vi "Emballage check code lu_MEDIC.vi"(0 "pièce en stock (testée et non emballée)":string[](array[string]), 1 "Quantité du lot de livraison":string="25", 2 "son code lu incorrect":path=path "\\\\Plz-inf-nas\\medic/PARAMETRES_TESTS/PROD_Data-Admin/Utopia - Erreur.WAV", 3 "n°commande":string="R03770/08-02.01.01", 5 "tableau des paramètres de la valve":string[](array[string])=["12-216C-04521 EQIFIL 104mA 230ohm", "1121058500", "AASSIIII", "25", "BPI", "n", "o"], 7 "tab pcs emballées historique":string[][](array[string]), 9 "chaîne lue par le lecteur IN":string="112105740008010105", 11 "tab pcs déjà emballées (histo+actu)":string[](array[string]), 12 "son code lu correct":path=path "\\\\Plz-inf-nas\\medic/PARAMETRES_TESTS/PROD_Data-Admin/lazer.wav", 13 "n° lot à scanner":string="****") -> (4 "largeur index":i16=4, 6 "Date production de la piéce":string="ZF", 8 "chaîne lue par le lecteur OUT":string="8411848-12ARZF-0005", 10 "Arrêter la série (T)":bool, 14 "offset sur code bar début index":i16=15, 15 "Paramètres OK(=> T)":bool=TRUE)   [LabVIEW 2020]
uses:
  Instance           3 31Saved   Emballage check code lu .vi
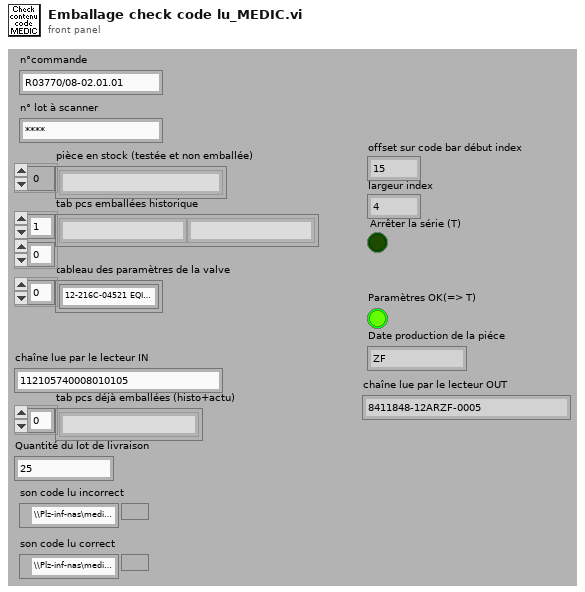
[diagram p1: front panel]
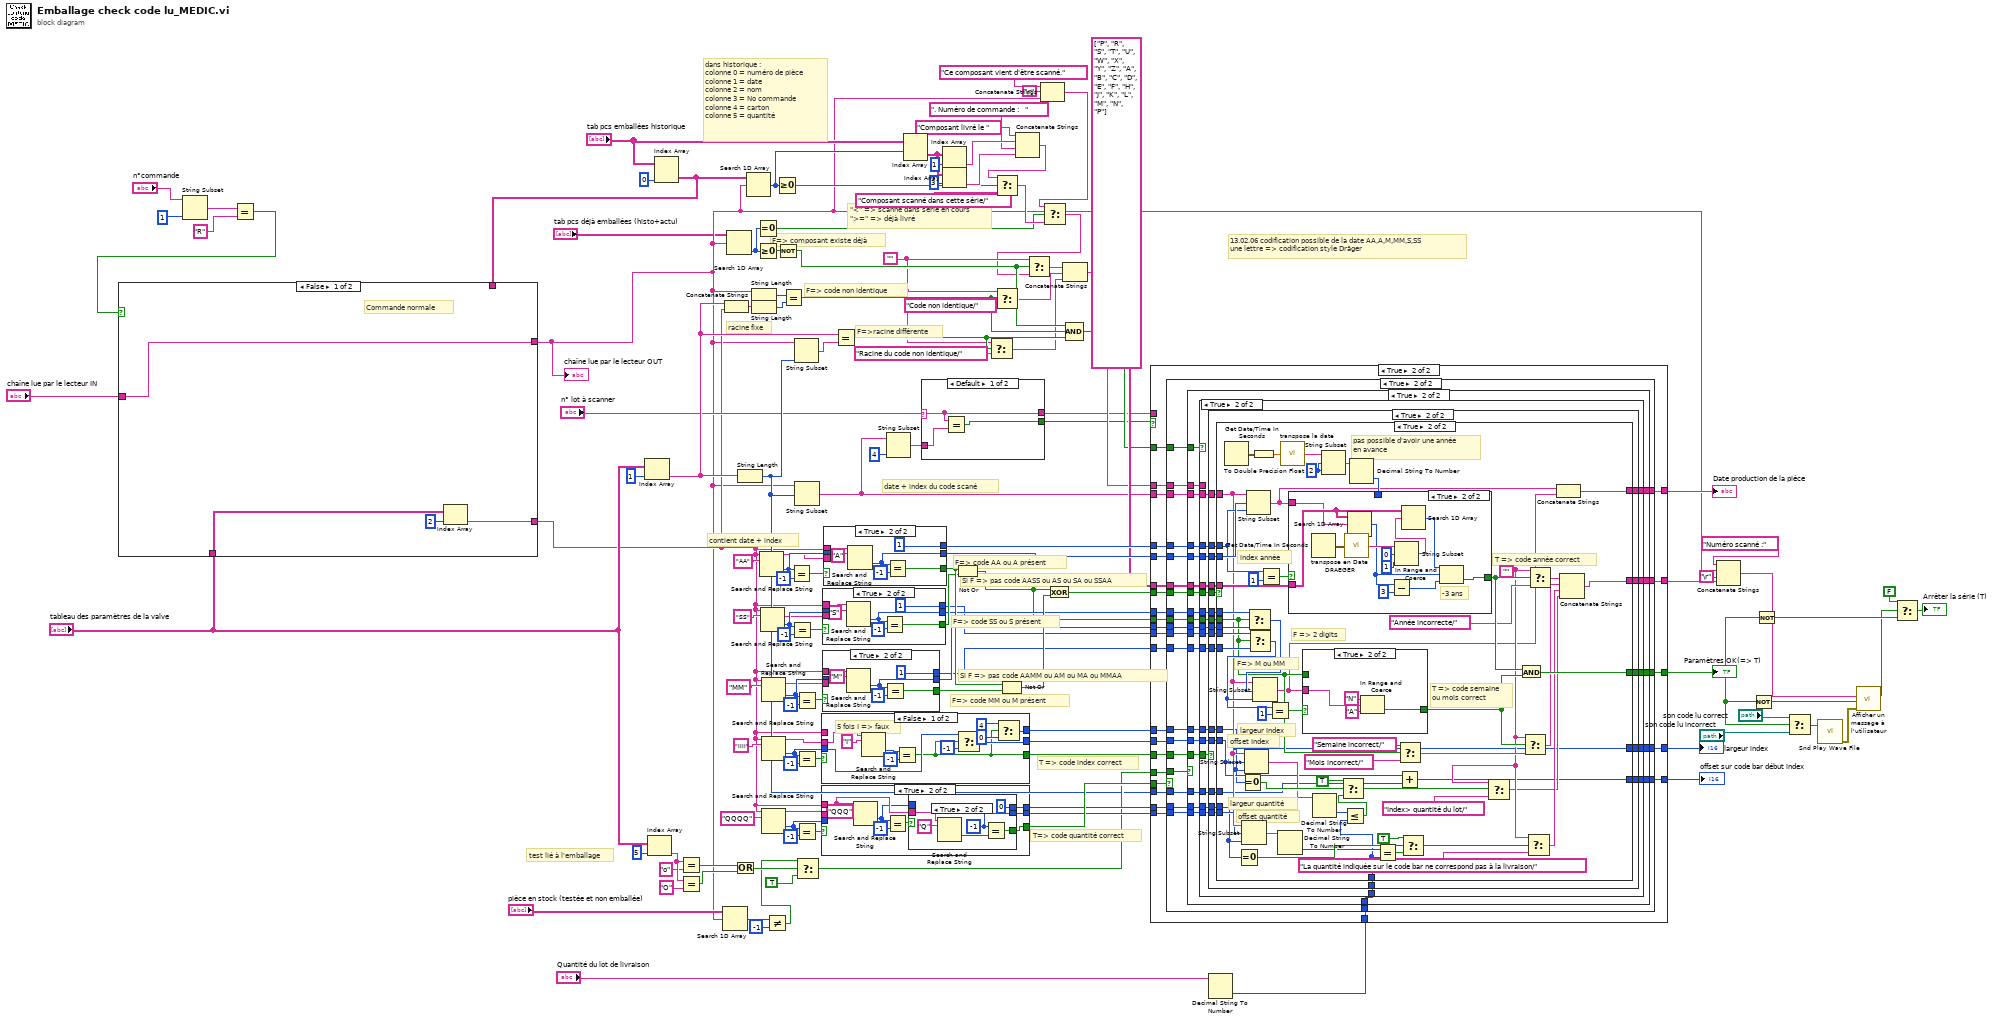
[diagram p0: block diagram]
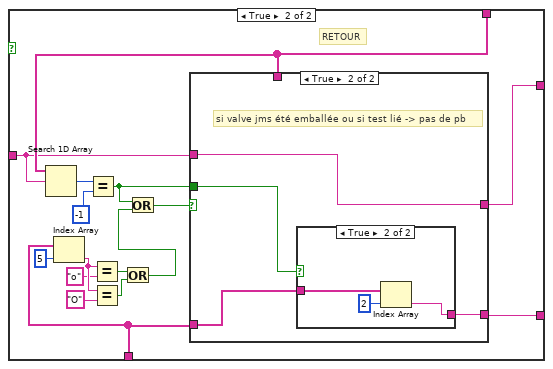
[diagram p2: hidden frame]
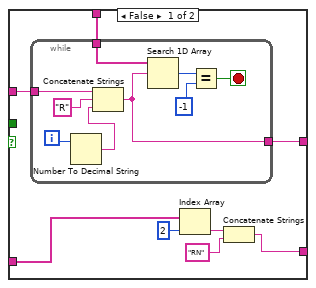
[diagram p3: hidden frame]
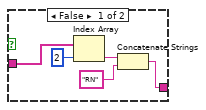
[diagram p4: hidden frame]
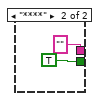
[diagram p5: hidden frame]
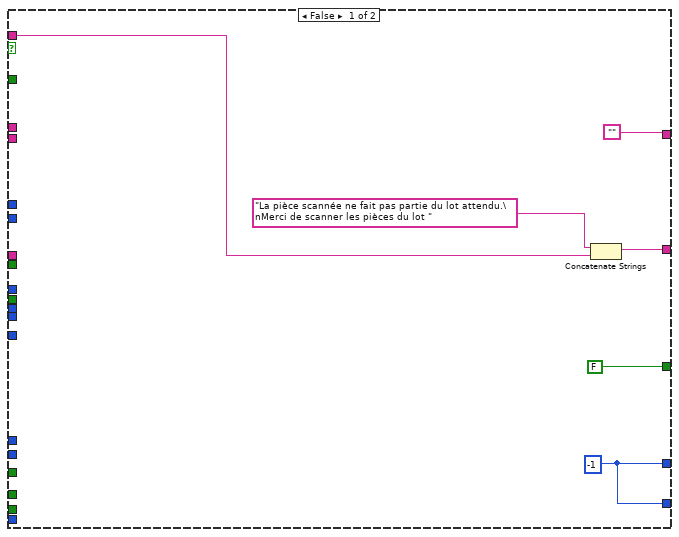
[diagram p6: hidden frame]
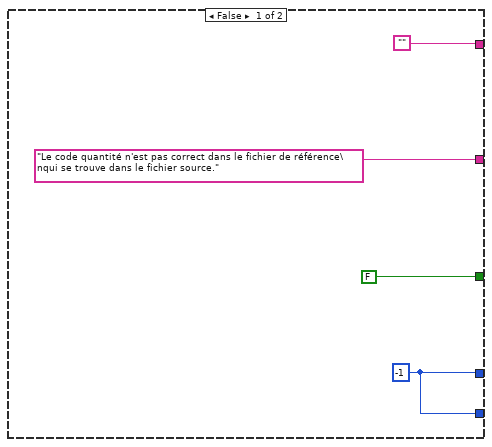
[diagram p7: hidden frame]
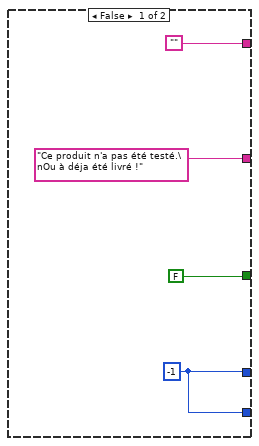
[diagram p8: hidden frame]
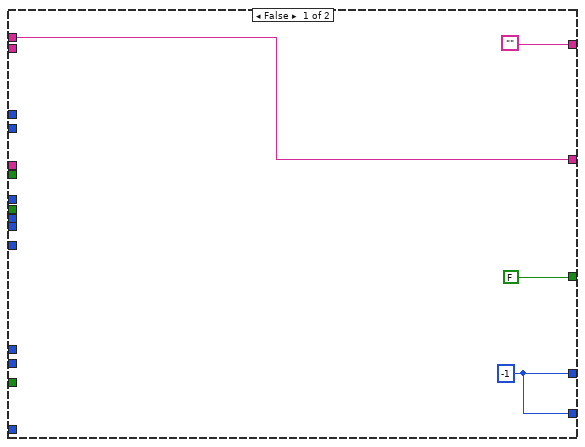
[diagram p9: hidden frame]
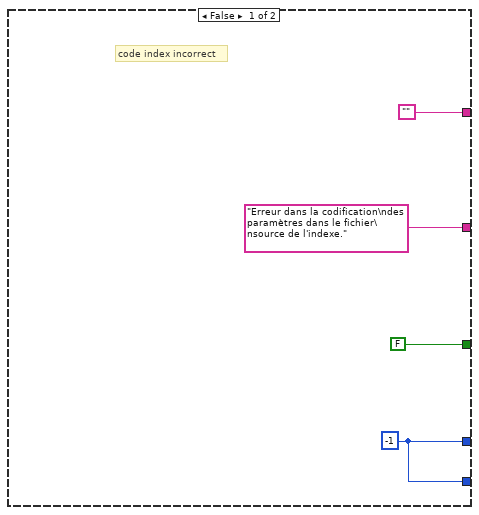
[diagram p10: hidden frame]
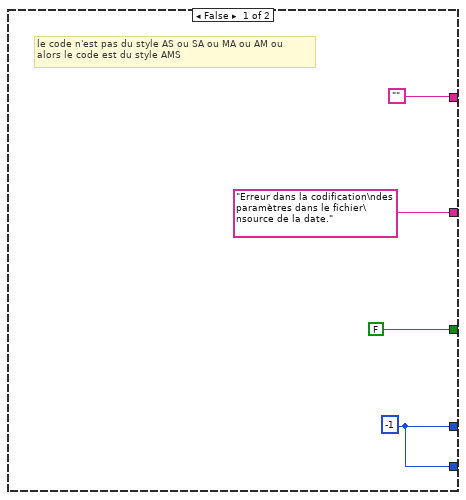
[diagram p11: hidden frame]
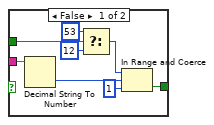
[diagram p12: hidden frame]
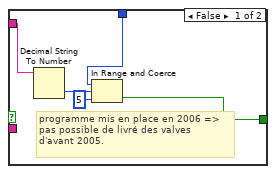
[diagram p13: hidden frame]
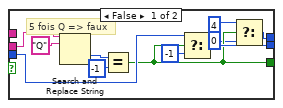
[diagram p14: hidden frame]
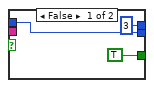
[diagram p15: hidden frame]
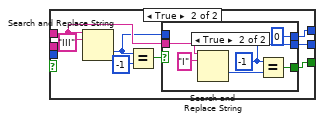
[diagram p16: hidden frame]
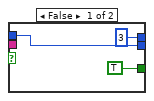
[diagram p17: hidden frame]
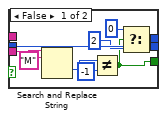
[diagram p18: hidden frame]
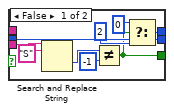
[diagram p19: hidden frame]
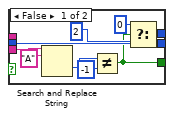
[diagram p20: hidden frame]
diagram:
  w91 = ""
  # "dans historique :\ncolonne 0 = numéro de pièce\ncolonne 1 = date\ncolonne 2 = nom\ncolonne 3 = No commande\ncolonne 4 = carton\ncolonne 5 = quantité"
  # "\"<\" => scanné dans série en cours\n\">=\" => déjà livré"
  # "T=> code quantité correct"
  # "test lié à l'emballage"
  # "Si F => pas code AASS ou AS ou SA ou SSAA"
  # "Si F => pas code AAMM ou AM ou MA ou MMAA"
  # "F=> code MM ou M présent"
  # "F=> code SS ou S présent"
  # "F=> code AA ou A présent"
  # "T => code index correct"
  # "13.02.06 codification possible de la date AA,A,M,MM,S,SS\nune lettre => codification style Dräger"
  # "date + index du code scané"
  # "contient date + index"
  # "racine fixe"
  # "F=> composant existe déjà"
  # "F=> code non identique"
  # "F=>racine différente"
  n1 = String Subset(string="n°commande", length (rest)=1 ("longueur (reste)")) -> (substring=w11:string)  [unwired: 1 in]
  n2 = Equal?(x=w11, y="R" ("expression régulière")) -> (x = y?=w10:bool)
  n3 = Index Array(array="tableau des paramètres de la valve", index=1) -> (element=w127:string)
  n4 = Index Array(array="tableau des paramètres de la valve", index=5) -> (element=w84:string)
  n5 = Index Array(array="tab pcs emballées historique", index (col)=0) -> (element=w1:string[])  [unwired: 1 in]
  n6 = case shown="False" w10 {
    tunnel: "chaîne lue par le lecteur IN" -> [w136 w149]
    tunnel: [w136 w148] -> w3
    tunnel: w1 -> [_ w150]
    tunnel: "tableau des paramètres de la valve" -> [w134 w138]
    tunnel: [w133 w139] -> w4
    frame False {
      # "Commande normale"
      n7 = Index Array(array=w134, index=2) -> (element=w133:string)
    }
    frame True {
      # "RETOUR"
      n8 = Search 1D Array(1D array=w150, element=w149) -> (index of element=w151:i32)  [unwired: 1 in]
      n9 = Index Array(array=w138, index=5) -> (element=w144:string)
      n10 = Equal?(x=w151, y=-1) -> (x = y?=w137:bool)
      n11 = Equal?(x=w144, y="o") -> (x = y?=w145:bool)
      n12 = Equal?(x=w144, y="O") -> (x = y?=w141:bool)
      n13 = Or(x=w145, y=w141) -> (x .or. y?=w140:bool)
      n14 = Or(x=w137, y=w140) -> (x .or. y?=w147:bool)
      n15 = case shown="True" w147 {
        tunnel: w150 -> [w160 _]
        tunnel: w149 -> [w159 w173]
        tunnel: [w158 w173] -> w148
        tunnel: [w154 w172] -> w139
        tunnel: w138 -> [w153 w171]
        tunnel: w137 -> [_ w170]
        frame False {
          n16 = while {
            tunnel: w160 -> [w168]
            tunnel: w159 -> [w167]
            tunnel: [w161] -> w158
            i -> [w165]
            stop <- w162 stop-if-true
            n17 = Number To Decimal String(number=w165) -> (decimal integer string=w166:string)  [unwired: 1 in]
            n18 = Concatenate Strings(w167, "R" ("expression régulière"), w166) -> (w161:string)
            n19 = Search 1D Array(1D array=w168, element=w161) -> (index of element=w164:i32)  [unwired: 1 in]
            n20 = Equal?(x=w164, y=-1) -> (x = y?=w162:bool)
          }
          n21 = Index Array(array=w153, index=2) -> (element=w156:string)
          n22 = Concatenate Strings(w156, "RN" ("chaîne")) -> (w154:string)
        }
        frame True {
          # "si valve jms été emballée ou si test lié -> pas de pb"
          n23 = case shown="True" w170 {
            tunnel: [w174 w180] -> w172
            tunnel: w171 -> [w177 w179]
            frame False {
              n24 = Index Array(array=w177, index=2) -> (element=w176:string)
              n25 = Concatenate Strings(w176, "RN" ("chaîne")) -> (w174:string)
            }
            frame True {
              n26 = Index Array(array=w179, index=2) -> (element=w180:string)
            }
          }
        }
      }
    }
  }
  "chaîne lue par le lecteur OUT" <- w3
  n27 = Equal?(x=w84, y="o") -> (x = y?=w85:bool)
  n28 = Equal?(x=w84, y="O") -> (x = y?=w81:bool)
  n29 = Search 1D Array(1D array="pièce en stock (testée et non emballée)", element=w3) -> (index of element=w62:i32)  [unwired: 1 in]
  n30 = Concatenate Strings(w127, w4) -> (w132:string)
  n31 = Search 1D Array(1D array="tab pcs déjà emballées (histo+actu)", element=w3) -> (index of element=w24:i32)  [unwired: 1 in]
  n32 = Or(x=w85, y=w81) -> (x .or. y?=w60:bool)
  n33 = String Length(string=w127) -> (length=w55:i32)
  n34 = Search 1D Array(1D array=w1, element=w3) -> (index of element=w25:i32)  [unwired: 1 in]
  n35 = String Length(string=w3) -> (length=w131:i32)
  n36 = String Length(string=w132) -> (length=w130:i32)
  n37 = Equal To 0?(x=w24) -> (x = 0?=w21:bool)
  n38 = Greater Or Equal To 0?(x=w24) -> (x >= 0?=w95:bool)
  n39 = Search and Replace String(input string=w4, search string="AA") -> (result string=w79:string, offset past replacement=w114:i32)  [unwired: 6 in, 2 out]
  n40 = Search and Replace String(input string=w4, search string="SS") -> (result string=w64:string, offset past replacement=w113:i32)  [unwired: 6 in, 2 out]
  n41 = Search and Replace String(input string=w4, search string="MM") -> (result string=w63:string, offset past replacement=w112:i32)  [unwired: 6 in, 2 out]
  n42 = Search and Replace String(input string=w4, search string="IIII") -> (result string=w80:string, offset past replacement=w73:i32)  [unwired: 6 in, 2 out]
  n43 = Search and Replace String(input string=w4, search string="QQQQ") -> (result string=w71:string, offset past replacement=w70:i32)  [unwired: 6 in, 2 out]
  n44 = Not Equal?(x=w62, y=-1) -> (x != y?=w56:bool)
  n45 = Greater Or Equal To 0?(x=w25) -> (x >= 0?=w31:bool)
  n46 = Not(x=w95) -> (.not. x?=w94:bool)
  n47 = Equal?(x=w131, y=w130) -> (x = y?=w96:bool)
  n48 = Equal?(x=w114, y=-1) -> (x = y?=w119:bool)
  n49 = Equal?(x=w113, y=-1) -> (x = y?=w120:bool)
  n50 = String Subset(string=w3, length (rest)=w55) -> (substring=w128:string)  [unwired: 1 in]
  n51 = String Subset(string=w3, offset (0)=w55) -> (substring=w14:string)  [unwired: 1 in]
  n52 = Equal?(x=w112, y=-1) -> (x = y?=w118:bool)
  n53 = Equal?(x=w73, y=-1) -> (x = y?=w115:bool)
  n54 = Equal?(x=w70, y=-1) -> (x = y?=w65:bool)
  n55 = Select(t=w56, s=w60, f=TRUE) -> (s? t:f=w58:bool)
  n56 = case shown="False" w115 {
    tunnel: w4 -> [_ w197]
    tunnel: [w183 w196] -> w74
    tunnel: w80 -> [w189 _]
    tunnel: w73 -> [w188 _]
    tunnel: [w186 w194] -> w72
    tunnel: [w182 w193] -> w67
    frame False {
      # "5 fois I => faux"
      n57 = Search and Replace String(input string=w189, search string="I") -> (offset past replacement=w190:i32)  [unwired: 6 in, 3 out]
      n58 = Equal?(x=w190, y=-1) -> (x = y?=w183:bool)
      n59 = Select(t=w188, s=w183, f=-1) -> (s? t:f=w186:i32)
      n60 = Select(t=4, s=w183, f=0) -> (s? t:f=w182:i32)
    }
    frame True {
      n61 = Search and Replace String(input string=w197, search string="III") -> (offset past replacement=w195:i32)  [unwired: 6 in, 3 out]
      n62 = Equal?(x=w195, y=-1) -> (x = y?=w198:bool)
      n63 = case shown="True" w198 {
        tunnel: w197 -> [_ w208]
        tunnel: [TRUE w206] -> w196
        tunnel: w195 -> [w202 _]
        tunnel: [w202 w205] -> w194
        tunnel: [3 0] -> w193
        frame False {
        }
        frame True {
          w205 = -1
          n64 = Search and Replace String(input string=w208, search string="I") -> (offset past replacement=w207:i32)  [unwired: 6 in, 3 out]
          n65 = Equal?(x=w205, y=w207) -> (x = y?=w206:bool)
        }
      }
    }
  }
  n66 = case shown="True" w65 {
    tunnel: w4 -> [_ w225]
    tunnel: [w213 w224] -> w69
    tunnel: w71 -> [w217 _]
    tunnel: w70 -> [w216 _]
    tunnel: [w214 w222] -> w68
    tunnel: [w210 w221] -> w66
    frame False {
      # "5 fois Q => faux"
      n67 = Search and Replace String(input string=w217, search string="Q") -> (offset past replacement=w218:i32)  [unwired: 6 in, 3 out]
      n68 = Equal?(x=w218, y=-1) -> (x = y?=w213:bool)
      n69 = Select(t=w216, s=w213, f=-1) -> (s? t:f=w214:i32)
      n70 = Select(t=4, s=w213, f=0) -> (s? t:f=w210:i32)
    }
    frame True {
      n71 = Search and Replace String(input string=w225, search string="QQQ") -> (offset past replacement=w223:i32)  [unwired: 6 in, 3 out]
      n72 = Equal?(x=w223, y=-1) -> (x = y?=w226:bool)
      n73 = case shown="True" w226 {
        tunnel: w225 -> [_ w236]
        tunnel: [TRUE w234] -> w224
        tunnel: w223 -> [w230 _]
        tunnel: [w230 w233] -> w222
        tunnel: [3 0] -> w221
        frame False {
        }
        frame True {
          w233 = -1
          n74 = Search and Replace String(input string=w236, search string="Q") -> (offset past replacement=w235:i32)  [unwired: 6 in, 3 out]
          n75 = Equal?(x=w233, y=w235) -> (x = y?=w234:bool)
        }
      }
    }
  }
  n76 = case shown="True" w118 {
    tunnel: w4 -> [_ w252]
    tunnel: [w239 w249] -> w111
    tunnel: [w246 w248] -> w103
    tunnel: w112 -> [w246 _]
    tunnel: [w241 1] -> w100
    tunnel: w63 -> [w242 _]
    frame False {
      n77 = Search and Replace String(input string=w242, search string="M") -> (offset past replacement=w245:i32)  [unwired: 6 in, 3 out]
      n78 = Not Equal?(x=w245, y=-1) -> (x != y?=w239:bool)
      n79 = Select(t=0, s=w239, f=2) -> (s? t:f=w241:i32)
    }
    frame True {
      n80 = Search and Replace String(input string=w252, search string="M") -> (offset past replacement=w248:i32)  [unwired: 6 in, 3 out]
      n81 = Equal?(x=w248, y=-1) -> (x = y?=w249:bool)
    }
  }
  n82 = case shown="True" w120 {
    tunnel: w4 -> [_ w267]
    tunnel: w113 -> [w261 _]
    tunnel: [w261 w264] -> w104
    tunnel: [w253 w263] -> w109
    tunnel: [w256 1] -> w101
    tunnel: w64 -> [w257 _]
    frame False {
      n83 = Search and Replace String(input string=w257, search string="S") -> (offset past replacement=w258:i32)  [unwired: 6 in, 3 out]
      n84 = Not Equal?(x=w258, y=-1) -> (x != y?=w253:bool)
      n85 = Select(t=0, s=w253, f=2) -> (s? t:f=w256:i32)
    }
    frame True {
      n86 = Search and Replace String(input string=w267, search string="S") -> (offset past replacement=w264:i32)  [unwired: 6 in, 3 out]
      n87 = Equal?(x=w264, y=-1) -> (x = y?=w263:bool)
    }
  }
  n88 = case shown="True" w119 {
    tunnel: w4 -> [_ w281]
    tunnel: w114 -> [w276 _]
    tunnel: [w276 w279] -> w106
    tunnel: [w268 w278] -> w110
    tunnel: [w271 1] -> w105
    tunnel: w79 -> [w274 _]
    frame False {
      n89 = Search and Replace String(input string=w274, search string="A") -> (offset past replacement=w272:i32)  [unwired: 6 in, 3 out]
      n90 = Not Equal?(x=w272, y=-1) -> (x != y?=w268:bool)
      n91 = Select(t=0, s=w268, f=2) -> (s? t:f=w271:i32)
    }
    frame True {
      n92 = Search and Replace String(input string=w281, search string="A") -> (offset past replacement=w279:i32)  [unwired: 6 in, 3 out]
      n93 = Equal?(x=w279, y=-1) -> (x = y?=w278:bool)
    }
  }
  n94 = Equal?(x=w127, y=w128) -> (x = y?=w97:bool)
  n95 = String Subset(string=w14, length (rest)=4 ("longueur (reste)")) -> (substring=w12:string)  [unwired: 1 in]
  n96 = Index Array(array="tab pcs emballées historique", index (row)=w25) -> (element=w35:string[])  [unwired: 1 in]
  n97 = case shown="Default" "n° lot à scanner" {
    selector: "n° lot à scanner" -> [w283 _]
    tunnel: [w285 TRUE] -> w16
    tunnel: [w283 "" ("n° lot à scanner")] -> w15
    tunnel: w12 -> [w284 _]
    frame Default {
      n98 = Equal?(x=w283, y=w284) -> (x = y?=w285:bool)
    }
    frame "****" {
    }
  }
  n99 = Index Array(array=w35, index=1) -> (element=w39:string)
  n100 = Index Array(array=w35, index=3) -> (element=w34:string)
  n101 = Not Or(1:w109, 2:w110) -> (0:w102:bool)
  n102 = Select(t=w91, s=w97, f="Racine du code non identique/") -> (s? t:f=w88:string)
  n103 = Select(t=w91, s=w96, f="Code non identique/") -> (s? t:f=w89:string)
  n104 = Not Or(1:w111, 2:w110) -> (0:w108:bool)
  n105 = Concatenate Strings("Composant livré le ", w39, ". Numéro de commande :   ", w34) -> (w37:string)
  n106 = Select(t=w37, s=w31, f="Composant scanné dans cette série/") -> (s? t:f=w22:string)
  n107 = Concatenate Strings("Ce composant vient d'être scanné.", "\r", w3) -> (w19:string)
  n108 = Select(t=w19, s=w21, f=w22) -> (s? t:f=w23:string)
  n109 = Select(t=w91, s=w94, f=w23) -> (s? t:f=w90:string)
  n110 = Exclusive Or(1:w108, 2:w102) -> (0:w107:bool)
  n111 = Concatenate Strings(w90, w89, w88) -> (w87:string)
  n112 = Compound Arithmetic op=AND(w94, w96, w97) -> (w98:bool)
  n113 = Decimal String To Number(string="Quantité du lot de livraison") -> (number=w76:i32)  [unwired: 2 in, 1 out]
  n114 = case shown="True" w16 {
    tunnel: w107 -> [_ w319]
    tunnel: w106 -> [_ w318]
    tunnel: w105 -> [_ w317]
    tunnel: w104 -> [_ w316]
    tunnel: w103 -> [_ w315]
    tunnel: w102 -> [_ w314]
    tunnel: w101 -> [_ w313]
    tunnel: w100 -> [_ w312]
    tunnel: w14 -> [_ w311]
    tunnel: string[] ["P", "R", "S", "T", "U", "W", "X", "Y", "Z", "A", "B", "C", "D", "E", "F", "H", "J", "K", "L", "M", "N", "P"] -> [_ w310]
    tunnel: w98 -> [_ w309]
    tunnel: w87 -> [_ w308]
    tunnel: w76 -> [_ w307]
    tunnel: w74 -> [_ w306]
    tunnel: w72 -> [_ w305]
    tunnel: w69 -> [_ w304]
    tunnel: w68 -> [_ w303]
    tunnel: w67 -> [_ w302]
    tunnel: w66 -> [_ w301]
    tunnel: w58 -> [_ w300]
    tunnel: w55 -> [_ w299]
    tunnel: [w288 w298] -> w54
    tunnel: [w288 w297] -> w53
    tunnel: [w291 w296] -> w47
    tunnel: ["" w295] -> w43
    tunnel: [FALSE w294] -> w29
    tunnel: w15 -> [w290 _]
    frame False {
      w288 = -1
      n115 = Concatenate Strings("La pièce scannée ne fait pas partie du lot attendu.\nMerci de scanner les pièces du lot ", w290) -> (w291:string)
    }
    frame True {
      n116 = case shown="True" w304 {
        tunnel: w306 -> [_ w348]
        tunnel: w319 -> [_ w347]
        tunnel: w318 -> [_ w346]
        tunnel: w317 -> [_ w345]
        tunnel: w316 -> [_ w344]
        tunnel: w315 -> [_ w343]
        tunnel: w314 -> [_ w342]
        tunnel: w313 -> [_ w341]
        tunnel: w312 -> [_ w340]
        tunnel: w311 -> [_ w339]
        tunnel: w310 -> [_ w338]
        tunnel: w309 -> [_ w337]
        tunnel: w308 -> [_ w336]
        tunnel: ["Le code quantité n'est pas correct dans le fichier de référence\nqui se trouve dans le fichier source." w335] -> w296
        tunnel: [FALSE w334] -> w294
        tunnel: w300 -> [_ w333]
        tunnel: w307 -> [_ w332]
        tunnel: w305 -> [_ w331]
        tunnel: w303 -> [_ w330]
        tunnel: w302 -> [_ w329]
        tunnel: w301 -> [_ w328]
        tunnel: ["" w327] -> w295
        tunnel: w299 -> [_ w326]
        tunnel: [w320 w325] -> w298
        tunnel: [w320 w324] -> w297
        frame False {
          w320 = -1
        }
        frame True {
          n117 = case shown="True" w333 {
            tunnel: w348 -> [_ w376]
            tunnel: w347 -> [_ w375]
            tunnel: w346 -> [_ w374]
            tunnel: w345 -> [_ w373]
            tunnel: w344 -> [_ w372]
            tunnel: w343 -> [_ w371]
            tunnel: w342 -> [_ w370]
            tunnel: w341 -> [_ w369]
            tunnel: w340 -> [_ w368]
            tunnel: w339 -> [_ w367]
            tunnel: w338 -> [_ w366]
            tunnel: w337 -> [_ w365]
            tunnel: w336 -> [_ w364]
            tunnel: ["Ce produit n'a pas été testé.\nOu à déja été livré !" w363] -> w335
            tunnel: [FALSE w362] -> w334
            tunnel: w332 -> [_ w361]
            tunnel: w331 -> [_ w360]
            tunnel: w330 -> [_ w359]
            tunnel: w329 -> [_ w358]
            tunnel: w328 -> [_ w357]
            tunnel: ["" w356] -> w327
            tunnel: w326 -> [_ w355]
            tunnel: [w349 w354] -> w325
            tunnel: [w349 w353] -> w324
            frame False {
              w349 = -1
            }
            frame True {
              n118 = case shown="True" w365 {
                tunnel: w376 -> [_ w402]
                tunnel: w375 -> [_ w401]
                tunnel: w374 -> [_ w400]
                tunnel: w373 -> [_ w399]
                tunnel: w372 -> [_ w398]
                tunnel: w371 -> [_ w397]
                tunnel: w370 -> [_ w396]
                tunnel: w369 -> [_ w395]
                tunnel: w368 -> [_ w394]
                tunnel: w367 -> [_ w393]
                tunnel: w366 -> [_ w392]
                tunnel: w364 -> [w380 _]
                tunnel: [w380 w390] -> w363
                tunnel: [FALSE w391] -> w362
                tunnel: w361 -> [_ w389]
                tunnel: w360 -> [_ w388]
                tunnel: w359 -> [_ w387]
                tunnel: w358 -> [_ w386]
                tunnel: w357 -> [_ w385]
                tunnel: ["" w384] -> w356
                tunnel: w355 -> [_ w383]
                tunnel: [w377 w382] -> w354
                tunnel: [w377 w381] -> w353
                frame False {
                  w377 = -1
                }
                frame True {
                  n119 = case shown="True" w402 {
                    tunnel: w401 -> [_ w427]
                    tunnel: w400 -> [_ w426]
                    tunnel: w399 -> [_ w425]
                    tunnel: w398 -> [_ w424]
                    tunnel: w397 -> [_ w423]
                    tunnel: w396 -> [_ w422]
                    tunnel: w395 -> [_ w421]
                    tunnel: w394 -> [_ w420]
                    tunnel: w393 -> [_ w419]
                    tunnel: w392 -> [_ w418]
                    tunnel: [FALSE w417] -> w391
                    tunnel: ["Erreur dans la codification\ndes paramètres dans le fichier\nsource de l'indexe." w416] -> w390
                    tunnel: w389 -> [_ w415]
                    tunnel: w388 -> [_ w414]
                    tunnel: w387 -> [_ w413]
                    tunnel: w386 -> [_ w412]
                    tunnel: w385 -> [_ w411]
                    tunnel: ["" w410] -> w384
                    tunnel: w383 -> [_ w409]
                    tunnel: [w403 w408] -> w382
                    tunnel: [w403 w407] -> w381
                    frame False {
                      w403 = -1
                      # "code index incorrect"
                    }
                    frame True {
                      n120 = case shown="True" w427 {
                        tunnel: w426 -> [_ w485]
                        tunnel: w425 -> [_ w477]
                        tunnel: w424 -> [_ w489]
                        tunnel: w423 -> [_ w488]
                        tunnel: w422 -> [_ w461]
                        tunnel: w421 -> [_ w487]
                        tunnel: w420 -> [_ w486]
                        tunnel: w419 -> [_ w457]
                        tunnel: w418 -> [_ w475]
                        tunnel: [FALSE w469] -> w417
                        tunnel: ["Erreur dans la codification\ndes paramètres dans le fichier\nsource de la date." w465] -> w416
                        tunnel: w415 -> [_ w444]
                        tunnel: w414 -> [_ w435]
                        tunnel: w413 -> [_ w456]
                        tunnel: w412 -> [_ w432]
                        tunnel: w411 -> [_ w455]
                        tunnel: ["" w436] -> w410
                        tunnel: w409 -> [_ w434]
                        tunnel: [w428 w433] -> w408
                        tunnel: [w428 w432] -> w407
                        frame False {
                          w428 = -1
                          # "le code n'est pas du style AS ou SA ou MA ou AM ou\nalors le code est du style AMS"
                        }
                        frame True {
                          w441 = ""
                          w482 = 2
                          # "largeur quantité"
                          # "largeur Index"
                          # "offset quantité"
                          # "offset Index"
                          # "T => code semaine\nou mois correct"
                          # "pas possible d'avoir une année\nen avance"
                          # "T => code année correct"
                          # "F=> M ou MM"
                          # "F => 2 digits"
                          # "index année"
                          n121 = Get Date/Time In Seconds() -> (seconds since 1Jan1904=w483:timestamp)
                          n122 = Equal To 0?(x=w455) -> (x = 0?=w454:bool)
                          n123 = Equal To 0?(x=w432) -> (x = 0?=w448:bool)
                          n124 = String Subset(string=w457, offset (0)=w456, length (rest)=w455) -> (substring=w450:string)
                          n125 = String Subset(string=w457, offset (0)=w435, length (rest)=w432) -> (substring=w446:string)
                          n126 = String Subset(string=w457, offset (0)=w485, length (rest)=w477) -> (substring=w438:string)
                          n127 = Select(t=w489, s=w461, f=w488) -> (s? t:f=w474:i32)
                          n128 = Select(t=w487, s=w461, f=w486) -> (s? t:f=w472:i32)
                          n129 = To Double Precision Float(number=w483) -> (double precision float=w484:dbl)
                          n130 = String Subset(string=w457, offset (0)=w474, length (rest)=w472) -> (substring=w437:string)
                          n131 = Equal?(x=w477, y=1) -> (x = y?=w476:bool)
                          n132 = Equal?(x=w472, y=1) -> (x = y?=w471:bool)
                          n133 = Decimal String To Number(string=w450) -> (number=w449:i32)  [unwired: 2 in, 1 out]
                          n134 = call "transpose la date.vi"("date a partir du 1 janvier 1904"=w484) -> ("Date:Semaine/année"=w481:string)
                          n135 = case shown="True" w471 {
                            tunnel: w437 -> [w497 w501]
                            tunnel: w461 -> [w493 _]
                            tunnel: [w490 w498] -> w467
                            frame False {
                              n136 = Decimal String To Number(string=w497) -> (number=w496:i32)  [unwired: 2 in, 1 out]
                              n137 = Select(t=53, s=w493, f=12) -> (s? t:f=w494:i32)
                              n138 = In Range and Coerce(upper limit=w494, x=w496, lower limit=1) -> (In Range?=w490:bool)  [unwired: 1 out]
                            }
                            frame True {
                              n139 = In Range and Coerce(upper limit="N", x=w501, lower limit="A") -> (In Range?=w498:bool)  [unwired: 1 out]
                            }
                          }
                          n140 = Decimal String To Number(string=w446) -> (number=w445:i32)  [unwired: 2 in, 1 out]
                          n141 = String Subset(string=w481, offset (0)=w482, length (rest)=w482) -> (substring=w480:string)
                          n142 = Less Or Equal?(x=w445, y=w444) -> (x <= y?=w443:bool)
                          n143 = Select(t=TRUE, s=w448, f=w443) -> (s? t:f=w442:bool)
                          n144 = Decimal String To Number(string=w480) -> (number=w479:i32)  [unwired: 2 in, 1 out]
                          n145 = case shown="True" w476 {
                            tunnel: w438 -> [w506 w508]
                            tunnel: w479 -> [w503 _]
                            tunnel: [w502 w516] -> w470
                            tunnel: w475 -> [_ w509]
                            frame False {
                              # "programme mis en place en 2006 =>\npas possible de livré des valves\nd'avant 2005."
                              n146 = Decimal String To Number(string=w506) -> (number=w505:i32)  [unwired: 2 in, 1 out]
                              n147 = In Range and Coerce(upper limit=w503, x=w505, lower limit=5) -> (In Range?=w502:bool)  [unwired: 1 out]
                            }
                            frame True {
                              # "-3 ans"
                              n148 = Get Date/Time In Seconds() -> (seconds since 1Jan1904=w514:timestamp)
                              n149 = call "transpose en Date DRAEGER.vi"("horodatage"=w514) -> ("Date Dräger"=w513:string)
                              n150 = Search 1D Array(1D array=w509, element=w508) -> (index of element=w507:i32)  [unwired: 1 in]
                              n151 = Subtract(x=w507, y=3) -> (x-y=w510:i32)
                              n152 = String Subset(string=w513, offset (0)=0, length (rest)=1) -> (substring=w512:string)
                              n153 = Search 1D Array(1D array=w509, element=w512) -> (index of element=w511:i32)  [unwired: 1 in]
                              n154 = In Range and Coerce(upper limit=w511, x=w507, lower limit=w510) -> (In Range?=w516:bool)  [unwired: 1 out]
                            }
                          }
                          n155 = Equal?(x=w449, y=w444) -> (x = y?=w451:bool)
                          n156 = Add(x=w435, y=w434) -> (x+y=w433:i32)
                          n157 = Select(t="Semaine incorrect/", s=w461, f="Mois incorrect/") -> (s? t:f=w464:string)
                          n158 = Select(t=TRUE, s=w454, f=w451) -> (s? t:f=w453:bool)
                          n159 = Select(t=w441, s=w442, f="Index> quantité du lot/") -> (s? t:f=w439:string)
                          n160 = And(x=w470, y=w467) -> (x .and. y?=w469:bool)
                          n161 = Select(t=w441, s=w467, f=w464) -> (s? t:f=w466:string)
                          n162 = Select(t=w441, s=w453, f="La quantité indiquée sur le code bar ne correspond pas à la livraison/") -> (s? t:f=w458:string)
                          n163 = Select(t=w441, s=w470, f="Année incorrecte/") -> (s? t:f=w468:string)
                          n164 = Concatenate Strings(w438, w437) -> (w436:string)
                          n165 = Concatenate Strings(w468, w466, w458, w439) -> (w465:string)
                        }
                      }
                    }
                  }
                }
              }
            }
          }
        }
      }
    }
  }
  "Paramètres OK(=> T)" <- w29
  "Date production de la piéce" <- w43
  "offset sur code bar début index" <- w54
  "largeur index" <- w53
  n166 = Concatenate Strings("Numéro scanné :", w3, "\r", w47) -> (w46:string)
  n167 = Not(x=w29) -> (.not. x?=w52:bool)
  n168 = Not(x=w29) -> (.not. x?=w51:bool)
  n169 = Select(t="son code lu correct", s=w29, f="son code lu incorrect") -> (s? t:f=w30:path)
  n170 = call <vilib>:"Snd Play Wave File.vi"("wave file path"=w30) -> ("error out"=w28:errorcluster)  [unwired: 9 in, 1 out]
  n171 = call "Afficher un message à l'utilisateur"("error in (no error)"=w28, "Enable"=w52, "Message"=w46) -> ("Continuer"=w48:bool)  [unwired: 7 in, 1 out]
  n172 = Select(t=FALSE, s=w48, f=w51) -> (s? t:f=→"Arrêter la série (T)":bool)
